vi "GetCalsFromFile.vi"() -> ()   [LabVIEW 2019]
uses:
  <vilib>/Utility/file.llb/Read Delimited Spreadsheet (string).vi
  <vilib>/Rock Robotics/Network Tables/NT Write String Array.vi
  GlobalVariableTest.vi
panel:
  out "element":string
  in  "Enum 2":T1(ring)
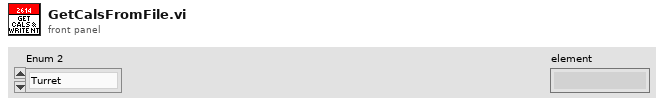
[diagram p1: front panel]
types:
  T1 = enum16{"Turret", "Magazine", "Intake", "Flywheel", "Drive", "Climb", "Control_Panel_"}
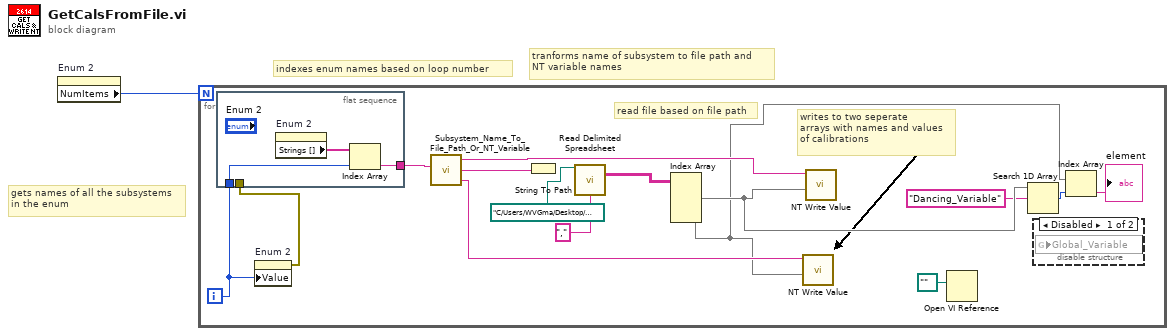
[diagram p0: block diagram]
diagram:
  # "tranforms name of subsystem to file path and\nNT variable names"
  # "indexes enum names based on loop number"
  # "gets names of all the subsystems\nin the enum"
  n1 = property on="Enum 2" class="Enum (strict)"() -> ("NumItems"=w1:u32)  [unwired: 2 in, 2 out]
  n2 = for {
    N: w1 -> [_]
    i -> [w11]
    # "writes to two seperate\narrays with names and values\nof calibrations"
    # "read file based on file path"
    n3 = flat-sequence {
      tunnel: w12 -> [_]
      tunnel: w11 -> [w18]
      tunnel: [w17] -> w10
      frame #0 {
        n4 = property on="Enum 2" class="Enum (strict)"() -> ("Strings []"=w19:string[])  [unwired: 2 in, 2 out]
        n5 = Index Array(array=w19, index=w18) -> (element=w17:string)
      }
    }
    n6 = property on="Enum 2" class="Enum (strict)"("Value"=w11) -> (error out=w12:errorcluster)  [unwired: 2 in, 1 out]
    n7 = call "Subsystem_Name_To_File_Path_Or_NT_Variable.vi"("Enum String Name"=w10) -> ("Names"=w14:string, "File Path"=w15:string, "Values"=w13:string)  [unwired: 5 in]
    n8 = String To Path(string=w15) -> ()  [unwired: 1 out]
    n9 = call-poly <vilib>:"Read Delimited Spreadsheet.vi"("file path (dialog if empty)"=path "C:/Users/WVGma/Desktop/TestCSV.csv", "delimiter (\\t)"="," ("delimiter (\\t)")) -> ("all rows"=w16:string[][])  [unwired: 8 in, 5 out]
    n10 = Index Array(array=w16) -> (element #1=w9:string[], element #2=w7:string[])  [unwired: 4 in]
    n11 = call-poly <vilib>:"NT Write Value.vi"("String Array"=w7, "Name"=w13) -> ()  [unwired: 9 in, 1 out]
    n12 = call-poly <vilib>:"NT Write Value.vi"("String Array"=w9, "Name"=w14) -> ()  [unwired: 9 in, 1 out]
    n13 = Open VI Reference(vi path=path "") -> ()  [unwired: 5 in, 2 out]
    n14 = Search 1D Array(1D array=w9, element="Dancing_Variable") -> (index of element=w8:i32)  [unwired: 1 in]
    n15 = disable-structure shown="Disabled" {
      frame Disabled {
        n16 = global read "GlobalVariableTest.vi" "Global_Variable"() -> ()  [unwired: 1 in]
      }
      frame Enabled {
      }
    }
    n17 = Index Array(array=w7, index=w8) -> (element=→"element":string)
  }
